vi "input waveform.vi"(1 "pulse parameters":T1={"Pe"=400.0, "dt"=0.001, "duty"=0.44999999999999996, "cycle time"=0.0, "Integration error"=0.0001, "cycles"=0} {"cycles" min=1; "cycle time" min=0.0; "duty" min=0.0 max=1.0; "dt" min=1e-12; "Pe" min=0.0}) -> (0 "input waveform":dbl[](array[numeric]))   [LabVIEW 2010]
uses:
  pulse parameters.ctl
  <vilib>/measure/NI_MABase.lvlib
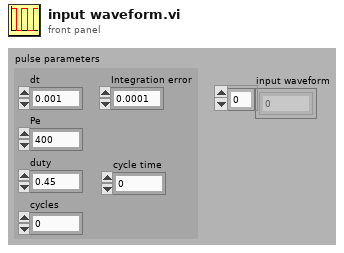
[diagram p1: front panel]
types:
  T1 = typedef "pulse parameters.ctl" = cluster{"Pe":dbl, "dt":dbl, "duty":dbl, "cycle time":dbl, "Integration error":dbl, "cycles":i16}
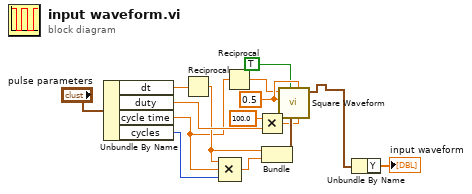
[diagram p0: block diagram]
diagram:
  w13 = 0.5 ("amplitude")
  n1 = Unbundle By Name("pulse parameters") -> ("dt"=w11:dbl, "duty"=w14:dbl, "cycle time"=w7:dbl, "cycles"=w8:i16)
  n2 = Reciprocal(x=w11) -> (1/x=w9:dbl)
  n3 = Compound Arithmetic op=MULTIPLY(w9, w7, w8) -> (w1:dbl)
  n4 = Reciprocal(x=w7) -> (1/x=w6:dbl)
  n5 = Multiply(x=100.0, y=w14) -> (x*y=w5:dbl)
  n6 = Bundle(w9, w1) -> (w10:cluster{dbl, dbl})  [unwired: 1 in]
  n7 = call <vilib>:"Square Waveform.vi"("duty cycle (%)"=w5, "offset"=w13, "sampling info"=w10, "reset signal"=TRUE, "amplitude"=w13, "frequency"=w6) -> ("signal out"=w3:waveform(dbl))  [unwired: 4 in, 1 out]
  n8 = Unbundle By Name(w3) -> ("Y"=→"input waveform":dbl[])
